vi "Unflatten FIFO Header and Extract Payload.vi"(7 "Extract Payload":bool=TRUE, 8 "error in (no error)":errorcluster, 9 "timeout in":bool, 10 "Buffer In":u8[](array[numeric]) format="%.0x", 11 "CIFChannels in":refnum<class "CIFChannels.lvclass">) -> (0 "error out":errorcluster, 1 "Header":T1, 2 "Payload":u8[](array[numeric]) format="%.0x", 3 "CIFChannels out":refnum<class "CIFChannels.lvclass">)   [LabVIEW 2021, in "CIFChannels.lvclass"]
uses:
  CIFChannels.lvclass
  CIFChannels.lvclass/CIFChannels.ctl
  ChannelCommon/ChannelCommon.lvlib
  ChannelCommon/typedef/FIFO Header.ctl
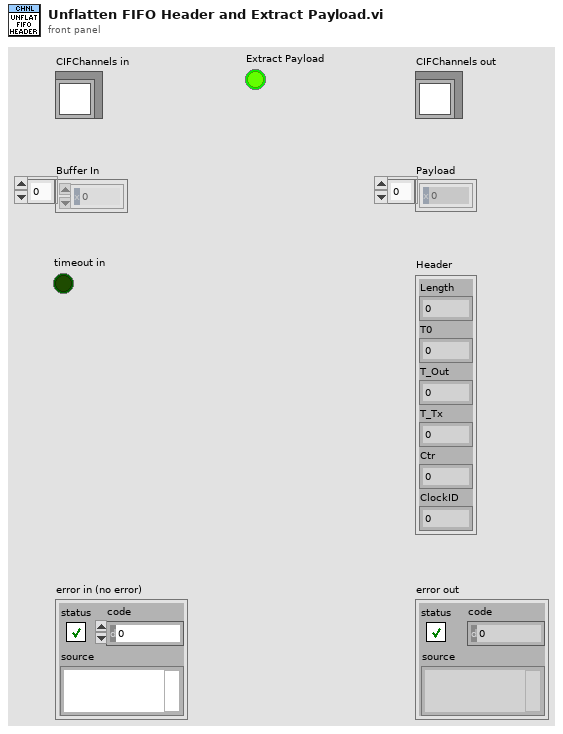
[diagram p1: front panel]
types:
  T1 = typedef "ChannelCommon.lvlib/FIFO Header.ctl" = cluster{"Length":u64, "T0":i64, "T_Out":i64, "T_Tx":i64, "Ctr":u64, "ClockID":u8}
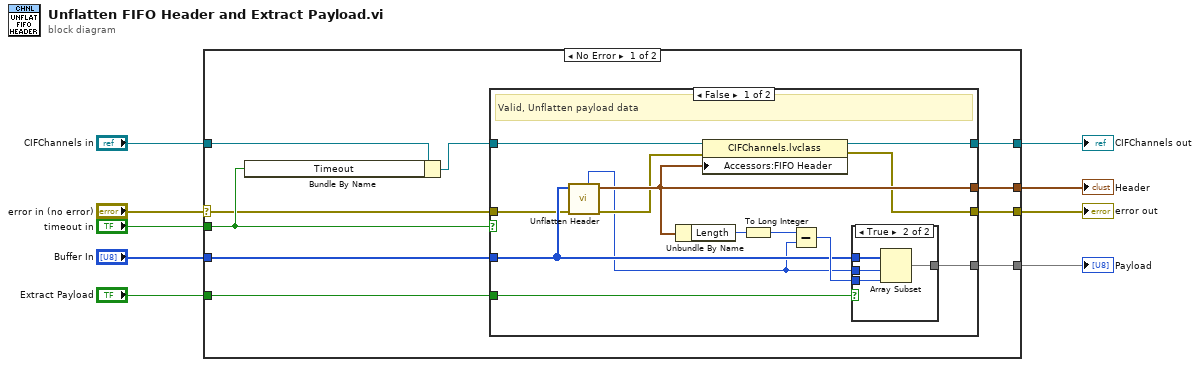
[diagram p0: block diagram]
diagram:
  n1 = case shown="No Error" "error in (no error)" {
    selector: "error in (no error)" -> [w12 w40]
    tunnel: [w15 w41] -> w5
    tunnel: "CIFChannels in" -> [w19 w41]
    tunnel: "timeout in" -> [w14 _]
    tunnel: [w17 _] -> w7
    tunnel: [w16 _] -> w8
    tunnel: "Buffer In" -> [w13 _]
    tunnel: [w11 w40] -> w2
    tunnel: "Extract Payload" -> [w10 _]
    frame No Error {
      n2 = Bundle By Name(cluster=w19, "Timeout"=w14) -> (w18:refnum<class "CIFChannels.lvclass">)
      n3 = case shown="False" w14 {
        tunnel: w18 -> [w32 w39]
        tunnel: [w29 _] -> w17
        tunnel: [w30 _] -> w16
        tunnel: [w31 w39] -> w15
        tunnel: w13 -> [w25 _]
        tunnel: w12 -> [w24 w38]
        tunnel: [w22 w38] -> w11
        tunnel: w10 -> [w21 _]
        frame False {
          # "Valid, Unflatten payload data"
          n4 = call "Unflatten Header.vi"("error in (no error)"=w24, "Flattened Data in"=w25) -> ("error out"=w23:errorcluster, "Header out"=w30:T1, "offset out"=w20:i32)  [unwired: 7 in]
          n5 = Unbundle By Name(w30) -> ("Length"=w28:u64)
          n6 = property class="CIFChannels.lvclass"(reference=w32, error in=w23, "Accessors:FIFO Header"=w30) -> (reference out=w31:refnum<class "CIFChannels.lvclass">, error out=w22:errorcluster)
          n7 = To Long Integer(number=w28) -> (32bit integer=w26:i32)
          n8 = Subtract(x=w26, y=w20) -> (x-y=w27:i32)
          n9 = case shown="True" w21 {
            tunnel: [w33 w37] -> w29
            tunnel: w20 -> [_ w36]
            tunnel: w27 -> [_ w35]
            tunnel: w25 -> [w33 w34]
            frame False {
            }
            frame True {
              n10 = Array Subset(array=w34, index=w36, length=w35) -> (w37:u8[])
            }
          }
        }
        frame True {
          # "Timeout"
        }
      }
    }
    frame Error {
    }
  }
  "error out" <- w2
  "CIFChannels out" <- w5
  "Header" <- w8
  "Payload" <- w7
